vi "Aimed_similarities.vi"() -> ()   [LabVIEW 2016]
panel:
  out "DistanceMatrixColorBox":u32[][](array[colorbox])=[[16777215, 16777215, 16777215, 16777215, 16777215, 16777215, 16777215, 16777215, 16777215, 16777215, 16777215, 16777215, 16777215, 16777215, 16777215, 16777215], [16777215, 16777215, 16777215, 16777215, 16777215, 16777215, 16777215, 16777215, 16777215, 16777215, 16777215, 16777215, 16777215, 16777215, 16777215, 16777215], [16777215, 16777215, 16777215, 16777215, 16777215, 16777215, 16777215, 16777215, 16777215, 16777215, 16777215, 16777215, 16777215, 16777215, 16777215, 16777215], [16777215, 16777215, 16777215, 16777215, 16777215, 16777215, 16777215, 16777215, 16777215, 16777215, 16777215, 16777215, 16777215, 16777215, 16777215, 16777215], [16777215, 16777215, 16777215, 16777215, 16777215, 16777215, 16777215, 16777215, 16777215, 16777215, 16777215, 16777215, 16777215, 16777215, 16777215, 16777215], [16777215, 16777215, 16777215, 16777215, 16777215, 16777215, 16777215, 16777215, 16777215, 16777215, 16777215, 16777215, 16777215, 16777215, 16777215, 16777215], [16777215, 16777215, 16777215, 16777215, 16777215, 16777215, 16777215, 16777215, 16777215, 16777215, 16777215, 16777215, 16777215, 16777215, 16777215, 16777215], [16777215, 16777215, 16777215, 16777215, 16777215, 16777215, 16777215, 16777215, 16777215, 16777215, 16777215, 16777215, 16777215, 16777215, 16777215, 16777215], [16777215, 16777215, 16777215, 16777215, 16777215, 16777215, 16777215, 16777215, 16777215, 16777215, 16777215, 16777215, 16777215, 16777215, 16777215, 16777215], [16777215, 16777215, 16777215, 16777215, 16777215, 16777215, 16777215, 16777215, 16777215, 16777215, 16777215, 16777215, 16777215, 16777215, 16777215, 16777215], [16777215, 16777215, 16777215, 16777215, 16777215, 16777215, 16777215, 16777215, 16777215, 16777215, 16777215, 16777215, 16777215, 16777215, 16777215, 16777215], [16777215, 16777215, 16777215, 16777215, 16777215, 16777215, 16777215, 16777215, 16777215, 16777215, 16777215, 16777215, 16777215, 16777215, 16777215, 16777215], [16777215, 16777215, 16777215, 16777215, 16777215, 16777215, 16777215, 16777215, 16777215, 16777215, 16777215, 16777215, 16777215, 16777215, 16777215, 16777215], [16777215, 16777215, 16777215, 16777215, 16777215, 16777215, 16777215, 16777215, 16777215, 16777215, 16777215, 16777215, 16777215, 16777215, 16777215, 16777215], [16777215, 16777215, 16777215, 16777215, 16777215, 16777215, 16777215, 16777215, 16777215, 16777215, 16777215, 16777215, 16777215, 16777215, 16777215, 16777215], [16777215, 16777215, 16777215, 16777215, 16777215, 16777215, 16777215, 16777215, 16777215, 16777215, 16777215, 16777215, 16777215, 16777215, 16777215, 16777215]]
  # "1"
  # "2"
  # "3"
  # "4"
  # "5"
  # "6"
  # "7"
  # "8"
  # "9"
  # "10"
  # "11"
  # "12"
  # "13"
  # "14"
  # "15"
  # "16"
  # "1"
  # "2"
  # "3"
  # "4"
  # "5"
  # "6"
  # "7"
  # "8"
  # "9"
  # "10"
  # "11"
  # "12"
  # "13"
  # "14"
  # "15"
  # "16"
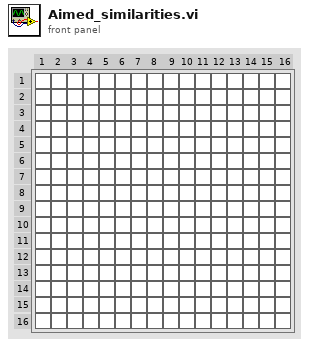
[diagram p1: front panel]
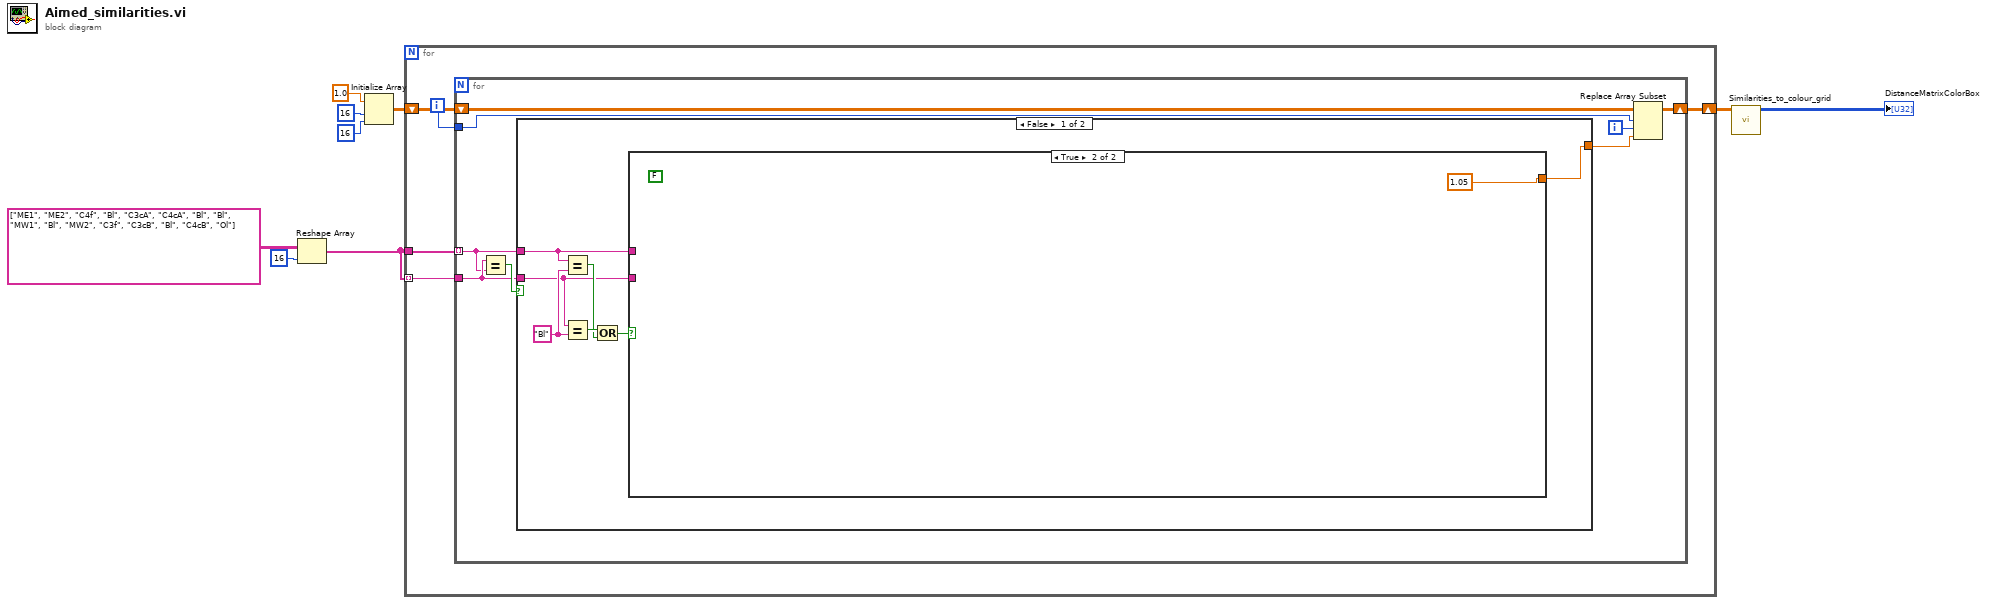
[diagram p0: block diagram]
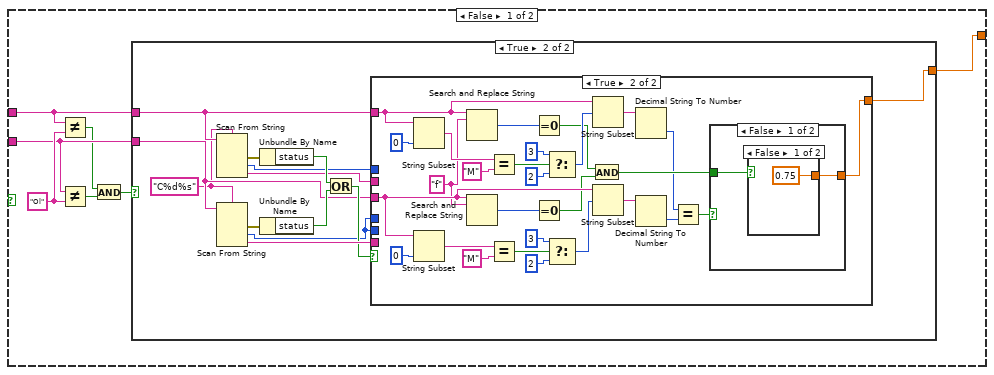
[diagram p2: hidden frame]
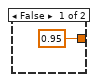
[diagram p3: hidden frame]
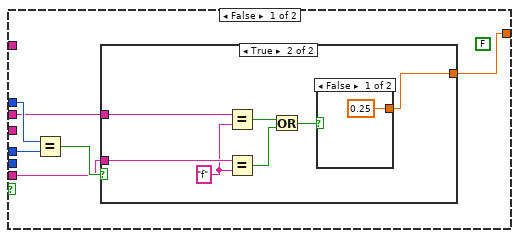
[diagram p4: hidden frame]
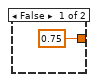
[diagram p5: hidden frame]
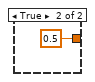
[diagram p6: hidden frame]
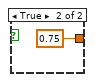
[diagram p7: hidden frame]
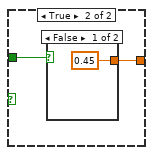
[diagram p8: hidden frame]
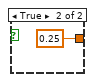
[diagram p9: hidden frame]
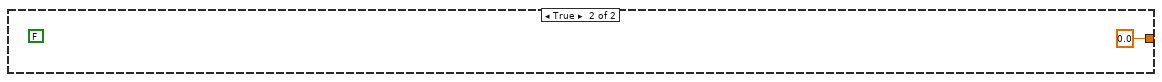
[diagram p10: hidden frame]
diagram:
  n1 = Reshape Array(string[][] [["ME1", "ME2", "C4f", "Bl"], ["C3cA", "C4cA", "Bl", "Bl"], ["MW1", "Bl", "MW2", "C3f"], ["C3cB", "Bl", "C4cB", "Ol"]], 16 ("dimension size")) -> (w4:string[])
  n2 = Initialize Array(1.0 ("element"), 16 ("dimension size"), 16 ("dimension size")) -> (w5:dbl[][])
  n3 = for {
    shift-right: [w12] -> w3
    shift-left: w5 -> [w13]
    tunnel: w4 -> [w14] mode=indexing
    tunnel: w4 -> [w11]
    i -> [w10]
    n4 = for {
      tunnel: w14 -> [w16]
      shift-right: [w19] -> w12
      shift-left: w13 -> [w20]
      tunnel: w11 -> [w15] mode=indexing
      tunnel: w10 -> [w22]
      i -> [w21]
      n5 = Equal?(x=w16, y=w15) -> (x = y?=w18:bool)
      n6 = case shown="False" w18 {
        tunnel: [w25 0.0 ("new element/subarray")] -> w17
        tunnel: w16 -> [w24 _]
        tunnel: w15 -> [w23 _]
        frame False {
          w28 = "Bl" ("y")
          n7 = Equal?(x=w23, y=w28) -> (x = y?=w26:bool)
          n8 = Equal?(x=w24, y=w28) -> (x = y?=w29:bool)
          n9 = Or(x=w29, y=w26) -> (x .or. y?=w27:bool)
          n10 = case shown="True" w27 {
            tunnel: [w36 1.05 ("new element/subarray")] -> w25
            tunnel: w24 -> [w33 _]
            tunnel: w23 -> [w35 _]
            frame False {
              w34 = "Ol" ("y")
              n11 = Not Equal?(x=w35, y=w34) -> (x != y?=w32:bool)
              n12 = Not Equal?(x=w33, y=w34) -> (x != y?=w31:bool)
              n13 = And(x=w32, y=w31) -> (x .and. y?=w30:bool)
              n14 = case shown="True" w30 {
                tunnel: [0.95 ("new element/subarray") w42] -> w36
                tunnel: w35 -> [_ w41]
                tunnel: w33 -> [_ w40]
                frame False {
                }
                frame True {
                  w39 = "C%d%s" ("format string")
                  n15 = Scan From String(format string=w39, input string=w41) -> (error out=w47:errorcluster, output 1=w44:i32, output 2=w43:string)  [unwired: 4 in, 2 out]
                  n16 = Scan From String(format string=w39, input string=w40) -> (error out=w49:errorcluster, output 1=w38:i32, output 2=w50:string)  [unwired: 4 in, 2 out]
                  n17 = Unbundle By Name(w47) -> ("status"=w45:bool)
                  n18 = Unbundle By Name(w49) -> ("status"=w48:bool)
                  n19 = Or(x=w45, y=w48) -> (x .or. y?=w46:bool)
                  n20 = case shown="True" w46 {
                    tunnel: w38 -> [w55 _]
                    tunnel: w50 -> [w51 _]
                    tunnel: w44 -> [w56 _]
                    tunnel: w43 -> [w52 _]
                    tunnel: [w53 w77] -> w42
                    tunnel: w41 -> [_ w75]
                    tunnel: w40 -> [_ w74]
                    tunnel: w38 -> [_ _]
                    frame False {
                      (unwired) FALSE
                      n21 = Equal?(x=w56, y=w55) -> (x = y?=w54:bool)
                      n22 = case shown="True" w54 {
                        tunnel: [0.75 ("new element/subarray") w58] -> w53
                        tunnel: w52 -> [_ w64]
                        tunnel: w51 -> [_ w63]
                        frame False {
                        }
                        frame True {
                          w62 = "f" ("y")
                          n23 = Equal?(x=w64, y=w62) -> (x = y?=w61:bool)
                          n24 = Equal?(x=w63, y=w62) -> (x = y?=w60:bool)
                          n25 = Or(x=w61, y=w60) -> (x .or. y?=w59:bool)
                          n26 = case shown="False" w59 {
                            tunnel: [0.25 0.5] -> w58
                            frame False {
                            }
                            frame True {
                            }
                          }
                        }
                      }
                    }
                    frame True {
                      w73 = "f" ("format string")
                      n27 = String Subset(string=w75, length (rest)=0 ("length (rest)")) -> (substring=w93:string)  [unwired: 1 in]
                      n28 = String Subset(string=w74, length (rest)=0 ("length (rest)")) -> (substring=w81:string)  [unwired: 1 in]
                      n29 = Search and Replace String(input string=w75, search string=w73) -> (number of replacements=w76:i32)  [unwired: 6 in, 3 out]
                      n30 = Search and Replace String(input string=w74, search string=w73) -> (number of replacements=w72:i32)  [unwired: 6 in, 3 out]
                      n31 = Equal?(x=w93, y="M") -> (x = y?=w91:bool)
                      n32 = Equal?(x=w81, y="M") -> (x = y?=w83:bool)
                      n33 = Equal To 0?(x=w76) -> (x = 0?=w71:bool)
                      n34 = Equal To 0?(x=w72) -> (x = 0?=w70:bool)
                      n35 = Select(t=3 ("offset (0)"), s=w91, f=2) -> (s? t:f=w88:i32)
                      n36 = Select(t=3 ("offset (0)"), s=w83, f=2) -> (s? t:f=w87:i32)
                      n37 = And(x=w71, y=w70) -> (x .and. y?=w69:bool)
                      n38 = String Subset(string=w75, offset (0)=w88) -> (substring=w67:string)  [unwired: 1 in]
                      n39 = String Subset(string=w74, offset (0)=w87) -> (substring=w84:string)  [unwired: 1 in]
                      n40 = Decimal String To Number(string=w67) -> (number=w68:i32)  [unwired: 2 in, 1 out]
                      n41 = Decimal String To Number(string=w84) -> (number=w79:i32)  [unwired: 2 in, 1 out]
                      n42 = Equal?(x=w68, y=w79) -> (x = y?=w78:bool)
                      n43 = case shown="False" w78 {
                        tunnel: [w96 w100] -> w77
                        tunnel: w69 -> [w95 w99]
                        frame False {
                          n44 = case shown="False" w95 {
                            tunnel: [0.75 ("new element/subarray") 0.75 ("new element/subarray")] -> w96
                            frame False {
                            }
                            frame True {
                            }
                          }
                        }
                        frame True {
                          n45 = case shown="False" w99 {
                            tunnel: [0.45 ("new element/subarray") 0.25 ("new element/subarray")] -> w100
                            frame False {
                            }
                            frame True {
                            }
                          }
                        }
                      }
                    }
                  }
                }
              }
            }
            frame True {
              (unwired) FALSE
            }
          }
        }
        frame True {
          (unwired) FALSE
        }
      }
      n46 = Replace Array Subset(array=w20, new element=w17, index (row)=w22, index (col)=w21) -> (w19:dbl[][])
    }
  }
  n47 = call "Similarities_to_colour_grid.vi"("Array in"=w3) -> ("Array out"=→"DistanceMatrixColorBox":u32[][])  [unwired: 10 in]
